vi "FFT.vi"() -> ()   [LabVIEW 2021]
uses:
  <userlib>/SciSDK/SciSDK_Labview.lvlib
panel:
  out "FFT Buffer Out":T1
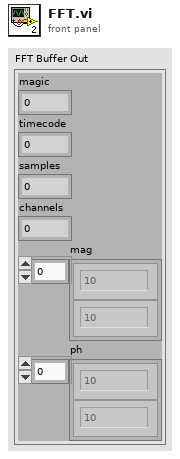
[diagram p1: front panel]
types:
  T1 = cluster{"magic":u32, "timecode":u32, "samples":u32, "channels":u32, "mag":dbl[], "ph":dbl[]}
  T2 = cluster{"Name":string, "Board Model":string, "Handle":u64}
  T3 = cluster{"Board Name":string, "Board Model":string, "Handle":u64}
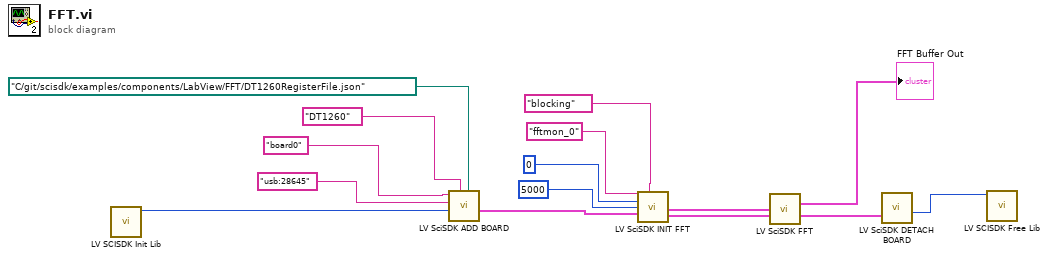
[diagram p0: block diagram]
diagram:
  n1 = call <userlib>:"LV SCISDK Init Lib.vi"() -> ("function return"=w15:u64)  [unwired: 11 in]
  n2 = call <userlib>:"LV SciSDK ADD BOARD.vi"("JsonFile"=path "C:/git/scisdk/examples/components/LabView/FFT/DT1260RegisterFile.json", "Board Model"="DT1260", "SciSDK Handle"=w15, "DevicePath"="usb:28645", "Name"="board0") -> ("Board Handle Out"=w10:T2)  [unwired: 4 in, 2 out]
  n3 = call <userlib>:"LV SciSDK INIT FFT.vi"("FFT Name"="fftmon_0", "Acq mode"="blocking", "Decimator"=u32 0, "Timeout"=5000, "Board Handle In"=w10) -> ("FFT Handle Out"=w4:cluster{"FFT Path":string, "FFT Name":string}, "Board Handle Out"=w5:T3)  [unwired: 8 in, 1 out]
  n4 = call <userlib>:"LV SciSDK FFT.vi"("FFT Handle In"=w4, "Board Handle In"=w5) -> ("FFT Buffer Out"=→"FFT Buffer Out":T1, "Board Handle Out"=w1:T3)  [unwired: 9 in, 3 out]
  n5 = call <userlib>:"LV SciSDK DETACH BOARD.vi"("Board Handle In"=w1) -> ("SciSDK Handle"=w2:u64)  [unwired: 9 in, 1 out]
  n6 = call <userlib>:"LV SCISDK Free Lib.vi"("handle"=w2) -> ()  [unwired: 9 in, 2 out]
